vi "SIM limit signal.vi"   [LabVIEW 2020]
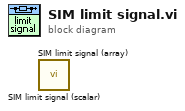
[diagram p0: block diagram]
diagram:
  n1 = call <vilib>:"SIM limit signal (scalar).vi"() -> ()  [unwired: 10 in, 2 out]
  n2 = call <vilib>:"SIM limit signal (array).vi"() -> ()  [unwired: 10 in, 2 out]
